vi "AlliGator Load FLIMbox Data v0.3.vi"(8 "Error In":errorcluster, 9 "Append":bool, 10 "FLIMbox Data in":T1 {"Base Frequency" min=-2147483648000000.0 max=2147483647000000.0}, 11 "File Path":path) -> (0 "Error Out":errorcluster, 2 "FLIMbox Data out":T1 {"Base Frequency" min=-2147483648000000.0 max=2147483647000000.0})   [LabVIEW 2021, in "AlliGator Files.lvlib"]
doc: "Loads FLIMBox dataset."
uses:
  AlliGator/AlliGator Files.lvlib
  FLIMbox Data.ctl
  FLIMbox Harmonic Data.ctl
  <vilib>/addons/h5labview2/base/lib_path.vi
  <vilib>/addons/h5labview2/base/H5Equery.vi
  <vilib>/addons/h5labview2/base/hid_t.ctl
  <vilib>/addons/h5labview2/dataset/H5Dread.llb/H5Dread.xnode
  <vilib>/addons/h5labview2/file/H5F.lvlib
  Time/Time.lvlib
  FLIMBox.lvlib
  <vilib>/addons/h5labview2/group/H5G.lvlib
panel:
  # "see the AlliGator License on the block diagram (Ctrl+E or Window:Show Block Diagram)"
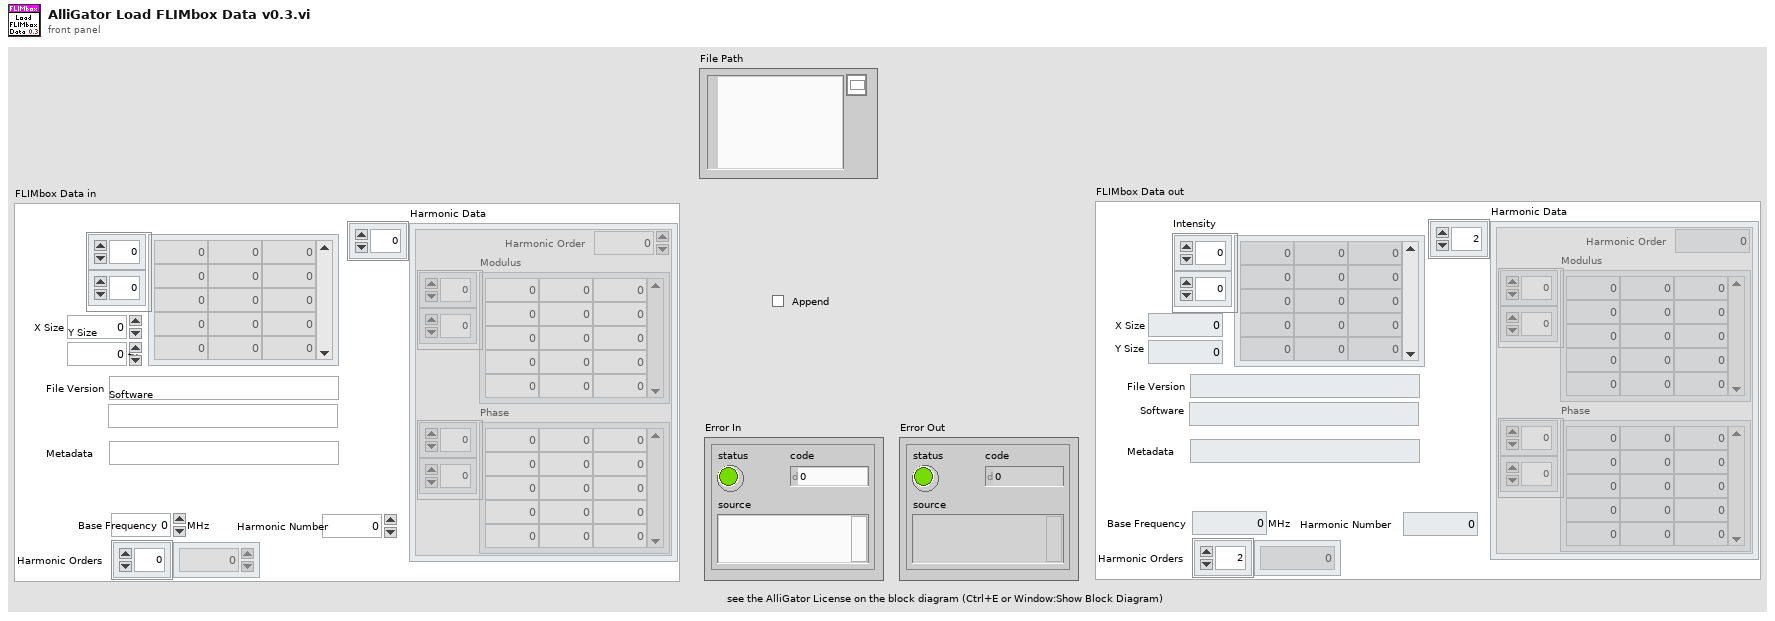
[diagram p1: front panel]
types:
  T1 = typedef "FLIMBox.lvlib/FLIMbox Data.ctl" = cluster{"Software":string, "Base Frequency":dbl[unit], "X Size":i32, "Y Size":i32, "Metadata":string, "Intensity":sgl[][], "Harmonic Number":u8, "Harmonic Orders":u8[], "Harmonic Data":T2[], "File Version":string}
  T2 = typedef "FLIMBox.lvlib/FLIMbox Harmonic Data.ctl" = cluster{"Modulus":sgl[][], "Phase":sgl[][], "Harmonic Order":u8}
  T3 = typedef "hid_t.ctl" = i64
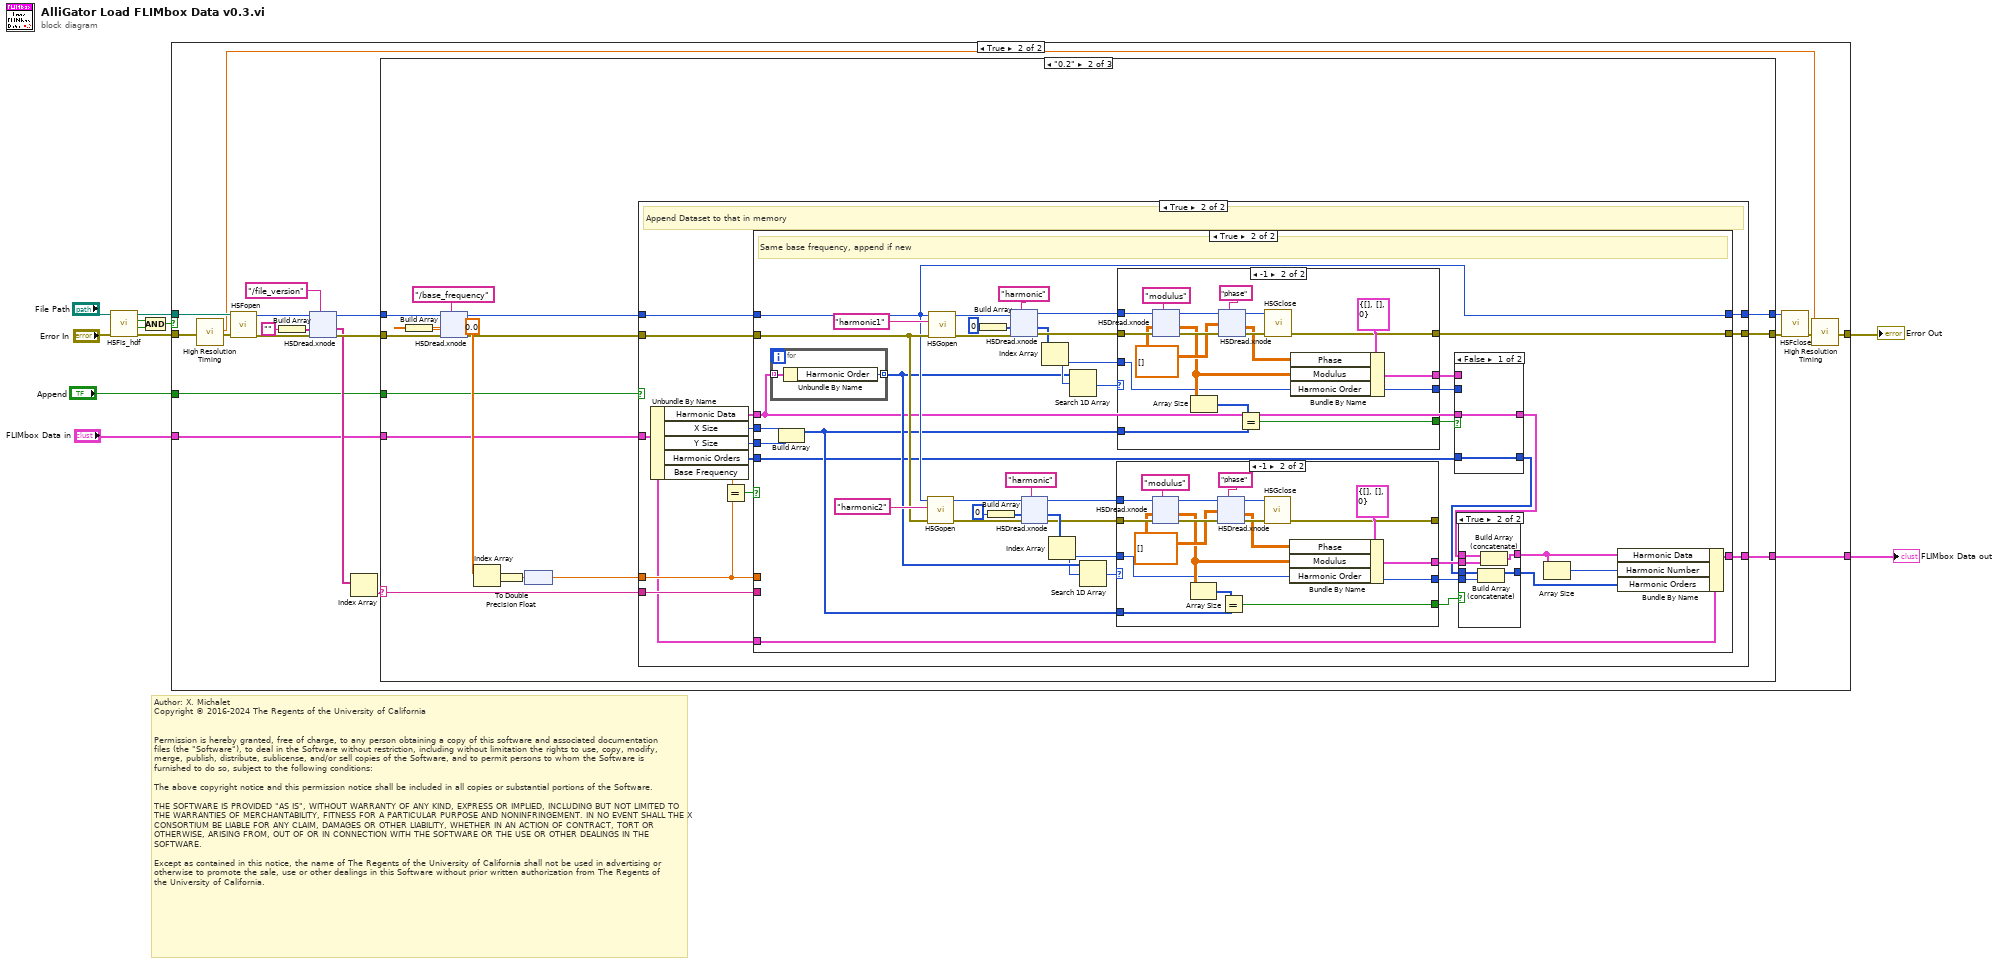
[diagram p0: block diagram]
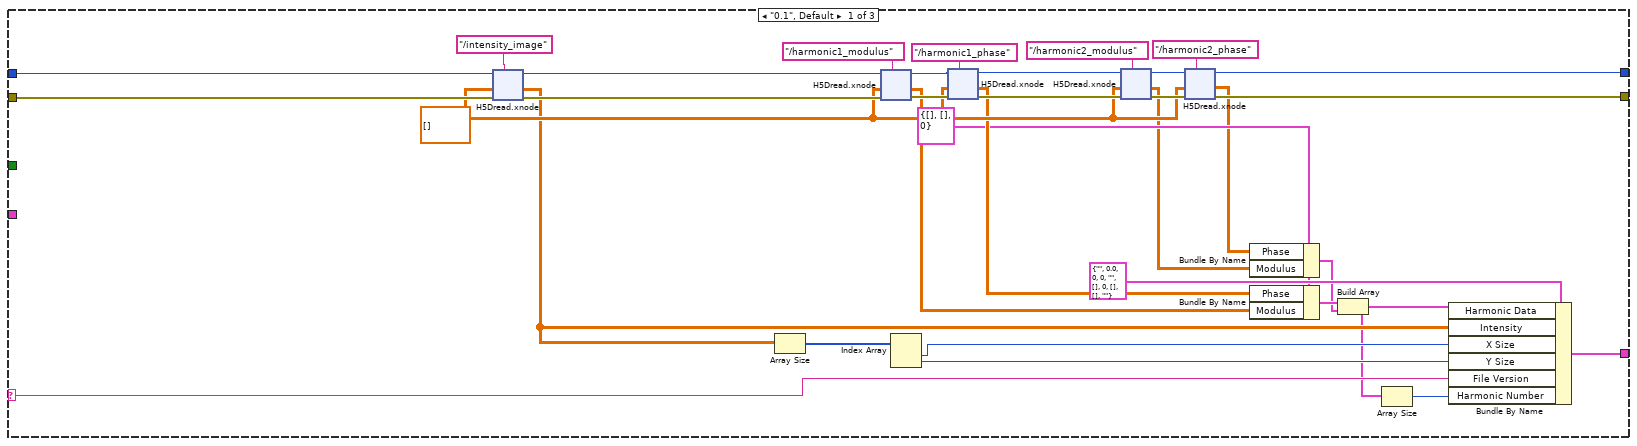
[diagram p3: hidden frame]
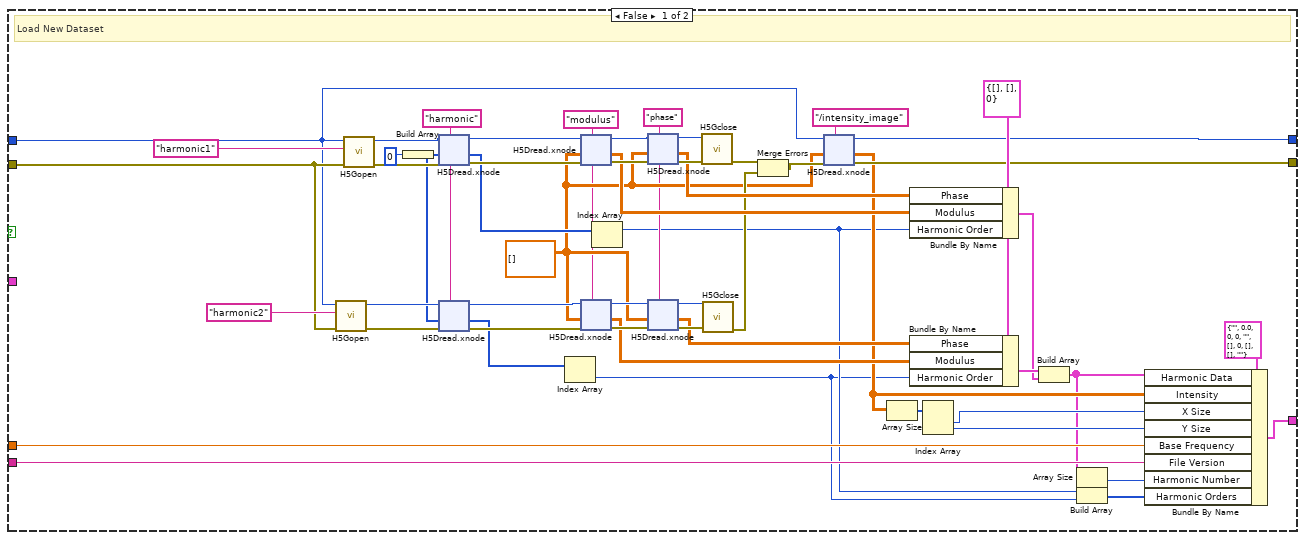
[diagram p4: hidden frame]
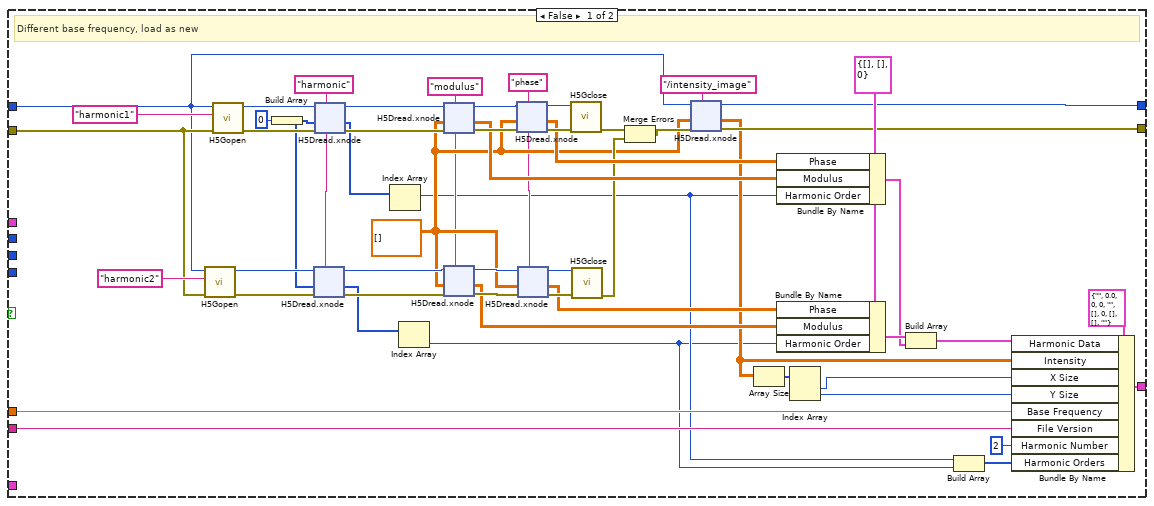
[diagram p5: hidden frame]
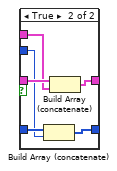
[diagram p7: hidden frame]
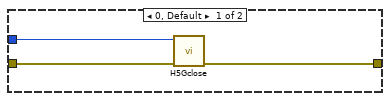
[diagram p8: hidden frame]
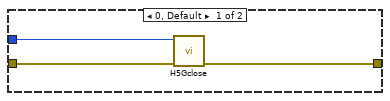
[diagram p9: hidden frame]
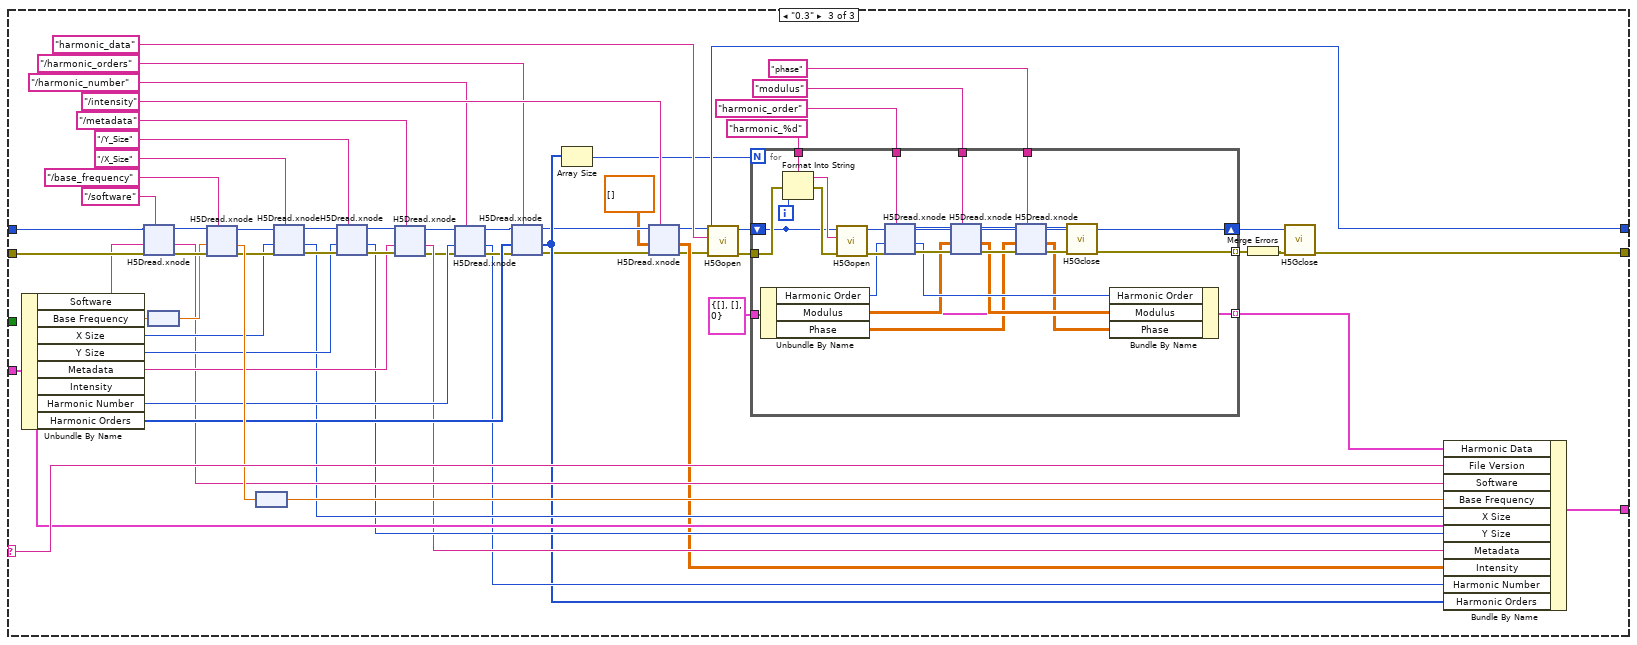
[diagram p10: hidden frame]
diagram:
  # "Author: X. Michalet\nCopyright © 2016-2024 The Regents of the University of California\n \n\nPermission is hereby granted, free of charge, to any person obtaining a copy of this software and associated documentation files (the \"Software\"), to deal in the Software without restriction, including without limitation the rights to use, copy, modify, merge, publish, distribute, sublicense, and/or sell copies of the Software, and to permit persons to whom the Software is furnished to do so, subject to the following conditions:\n\nThe above copyright notice and this permission notice shall be included in all copies or substantial portions of the Software.\n\nTHE SOFTWARE IS PROVIDED \"AS IS\", WITHOUT WARRANTY OF ANY KIND, EXPRESS OR IMPLIED, INCLUDING BUT NOT LIMITED TO THE WARRANTIES OF MERCHANTABILITY, FITNESS FOR A PARTICULAR PURPOSE AND NONINFRINGEMENT. IN NO EVENT SHALL THE X CONSORTIUM BE LIABLE FOR ANY CLAIM, DAMAGES OR OTHER LIABILITY, WHETHER IN AN ACTION OF CONTRACT, TORT OR OTHERWISE, ARISING FROM, OUT OF OR IN CONNECTION WITH THE SOFTWARE OR THE USE OR OTHER DEALINGS IN THE SOFTWARE.\n\nExcept as contained in this notice, the name of The Regents of the University of California shall not be used in advertising or otherwise to promote the sale, use or other dealings in this Software without prior written authorization from The Regents of the University of California."
  n1 = call <vilib>:"H5Fis_hdf.vi"("error in (no error)"="Error In", "path in"="File Path") -> ("error out"=w5:errorcluster, "valid?"=w10:bool, "exists?"=w11:bool, "path out"=w6:path)  [unwired: 6 in]
  n2 = And(x=w11, y=w10) -> (x .and. y?=w7:bool)
  n3 = case shown="True" w7 {
    tunnel: w6 -> [_ w31]
    tunnel: w5 -> [w12 w30]
    tunnel: [w12 w19] -> w4
    tunnel: [_ w20] -> w3
    tunnel: "FLIMbox Data in" -> [_ w14]
    tunnel: "Append" -> [_ w13]
    frame False {
    }
    frame True {
      n4 = call "High Resolution Timing.vi"("Error In"=w30) -> ("elapsed (relative) seconds"=w18:dbl, "Error Out"=w32:errorcluster)  [unwired: 16 in, 1 out]
      n5 = call <vilib>:"H5Fopen.vi"("error in (no error)"=w32, "path"=w31) -> ("error out"=w24:errorcluster, "ref out"=w29:T3)  [unwired: 8 in]
      n6 = Build Array("") -> (w17:string[])
      n7 = xnode "H5Dread.xnode"("dataset name (this)"="/file_version", "error in (no error)"=w24, "default"=w17, "ref in"=w29) -> ("error out"=w25:errorcluster, "data"=w15:string[], "ref out"=w26:T3)  [unwired: 2 in, 1 out]
      n8 = Index Array(array=w15) -> (element=w16:string)  [unwired: 1 in]
      n9 = case shown="\"0.2\"" w16 {
        selector: w16 -> [w57 w172 w773]
        tunnel: w26 -> [w81 w170 w769]
        tunnel: w25 -> [w79 w171 w768]
        tunnel: [w65 w162 w724] -> w23
        tunnel: [w64 w160 w717] -> w21
        tunnel: [w58 w173 w774] -> w20
        tunnel: w14 -> [_ w158 w741]
        tunnel: w13 -> [_ w159 _]
        frame "0.1", Default {
          w54 = T2 {"Modulus"=[], "Phase"=[], "Harmonic Order"=0} ("Harmonic Data")
          w66 = sgl[][] [] ("Data")
          n10 = xnode "H5Dread.xnode"("dataset name (this)"="/intensity_image", "error in (no error)"=w79, "default"=w66, "ref in"=w81) -> ("error out"=w78:errorcluster, "data"=w62:sgl[][], "ref out"=w77:T3)  [unwired: 2 in, 1 out]
          n11 = Array Size(array=w62) -> (size(s)=w61:i32[])
          n12 = xnode "H5Dread.xnode"("dataset name (this)"="/harmonic1_modulus", "error in (no error)"=w78, "default"=w66, "ref in"=w77) -> ("error out"=w74:errorcluster, "data"=w56:sgl[][], "ref out"=w75:T3)  [unwired: 2 in, 1 out]
          n13 = Index Array(array=w61) -> (element #1=w60:i32, element #2=w59:i32)  [unwired: 2 in]
          n14 = xnode "H5Dread.xnode"("dataset name (this)"="/harmonic1_phase", "error in (no error)"=w74, "default"=w66, "ref in"=w75) -> ("error out"=w68:errorcluster, "data"=w55:sgl[][], "ref out"=w67:T3)  [unwired: 2 in, 1 out]
          n15 = xnode "H5Dread.xnode"("dataset name (this)"="/harmonic2_modulus", "error in (no error)"=w68, "default"=w66, "ref in"=w67) -> ("error out"=w71:errorcluster, "data"=w52:sgl[][], "ref out"=w70:T3)  [unwired: 2 in, 1 out]
          n16 = xnode "H5Dread.xnode"("dataset name (this)"="/harmonic2_phase", "error in (no error)"=w71, "default"=w66, "ref in"=w70) -> ("error out"=w65:errorcluster, "data"=w53:sgl[][], "ref out"=w64:T3)  [unwired: 2 in, 1 out]
          n17 = Bundle By Name(cluster=w54, "Phase"=w53, "Modulus"=w52) -> (w50:T2)
          n18 = Bundle By Name(cluster=w54, "Phase"=w55, "Modulus"=w56) -> (w51:T2)
          n19 = Build Array(w51, w50) -> (w49:T2[])
          n20 = Array Size(array=w49) -> (size(s)=w48:i32)
          n21 = Bundle By Name(cluster=T1 {"Software"="", "Base Frequency"=0.0, "X Size"=0, "Y Size"=0, "Metadata"="", "Intensity"=[], "Harmonic Number"=0, "Harmonic Orders"=[], "Harmonic Data"=[], "File Version"=""} ("Data"), "Harmonic Data"=w49, "Intensity"=w62, "X Size"=w60, "Y Size"=w59, "File Version"=w57, "Harmonic Number"=w48) -> (w58:T1)
        }
        frame "0.2" {
          n22 = Build Array(sgl 0.0 ("U32")) -> (w165:sgl[])
          n23 = xnode "H5Dread.xnode"("dataset name (this)"="/base_frequency", "error in (no error)"=w171, "default"=w165, "ref in"=w170) -> ("error out"=w163:errorcluster, "data"=w167:sgl[], "ref out"=w161:T3)  [unwired: 2 in, 1 out]
          n24 = Index Array(array=w167) -> (element=w164:sgl)  [unwired: 1 in]
          n25 = To Double Precision Float(number=w164) -> (double precision float=w157:dbl)
          n26 = node(w157) -> (w166:dbl[unit])
          n27 = case shown="True" w159 {
            tunnel: [w234 w361] -> w173
            tunnel: w172 -> [w233 w360]
            tunnel: w166 -> [w229 w354]
            tunnel: w163 -> [w205 w359]
            tunnel: [w203 w358] -> w162
            tunnel: w161 -> [w201 w357]
            tunnel: [w200 w356] -> w160
            tunnel: w158 -> [_ w349]
            frame False {
              w194 = "harmonic" ("dataset name (this)")
              w232 = T2 {"Modulus"=[], "Phase"=[], "Harmonic Order"=0} ("Harmonic Data")
              w196 = "phase" ("dataset name (this)")
              w195 = "modulus" ("dataset name (this)")
              w199 = sgl[][] [] ("Data")
              # "Load New Dataset"
              n28 = call <vilib>:"H5Gopen.vi"("error in (no error)"=w205, "name"="harmonic2" ("dataset name (this)"), "ref in"=w201) -> ("error out"=w213:errorcluster, "group out"=w212:T3)  [unwired: 7 in]
              n29 = call <vilib>:"H5Gopen.vi"("error in (no error)"=w205, "name"="harmonic1" ("dataset name (this)"), "ref in"=w201) -> ("error out"=w220:errorcluster, "group out"=w219:T3)  [unwired: 7 in]
              n30 = Build Array(u8 0 ("Harmonic Order")) -> (w197:u8[])
              n31 = xnode "H5Dread.xnode"("dataset name (this)"=w194, "error in (no error)"=w220, "default"=w197, "ref in"=w219) -> ("error out"=w228:errorcluster, "data"=w225:u8[], "ref out"=w227:T3)  [unwired: 2 in, 1 out]
              n32 = xnode "H5Dread.xnode"("dataset name (this)"=w194, "error in (no error)"=w213, "default"=w197, "ref in"=w212) -> ("error out"=w224:errorcluster, "data"=w222:u8[], "ref out"=w223:T3)  [unwired: 2 in, 1 out]
              n33 = Index Array(array=w222) -> (element=w190:u8)  [unwired: 1 in]
              n34 = xnode "H5Dread.xnode"("dataset name (this)"=w195, "error in (no error)"=w228, "default"=w199, "ref in"=w227) -> ("error out"=w241:errorcluster, "data"=w215:sgl[][], "ref out"=w242:T3)  [unwired: 2 in, 1 out]
              n35 = xnode "H5Dread.xnode"("dataset name (this)"=w195, "error in (no error)"=w224, "default"=w199, "ref in"=w223) -> ("error out"=w240:errorcluster, "data"=w206:sgl[][], "ref out"=w239:T3)  [unwired: 2 in, 1 out]
              n36 = Index Array(array=w225) -> (element=w191:u8)  [unwired: 1 in]
              n37 = xnode "H5Dread.xnode"("dataset name (this)"=w196, "error in (no error)"=w241, "default"=w199, "ref in"=w242) -> ("error out"=w218:errorcluster, "data"=w216:sgl[][], "ref out"=w217:T3)  [unwired: 2 in, 1 out]
              n38 = xnode "H5Dread.xnode"("dataset name (this)"=w196, "error in (no error)"=w240, "default"=w199, "ref in"=w239) -> ("error out"=w210:errorcluster, "data"=w207:sgl[][], "ref out"=w211:T3)  [unwired: 2 in, 1 out]
              n39 = call <vilib>:"H5Gclose.vi"("error in (no error)"=w218, "group in"=w217) -> ("error out"=w209:errorcluster)  [unwired: 9 in]
              n40 = call <vilib>:"H5Gclose.vi"("error in (no error)"=w210, "group in"=w211) -> ("error out"=w208:errorcluster)  [unwired: 9 in]
              n41 = Merge Errors(w209, w208) -> (w204:errorcluster)
              n42 = xnode "H5Dread.xnode"("dataset name (this)"="/intensity_image", "error in (no error)"=w204, "default"=w199, "ref in"=w201) -> ("error out"=w203:errorcluster, "data"=w198:sgl[][], "ref out"=w200:T3)  [unwired: 2 in, 1 out]
              n43 = Array Size(array=w198) -> (size(s)=w237:i32[])
              n44 = Bundle By Name(cluster=w232, "Phase"=w216, "Modulus"=w215, "Harmonic Order"=w191) -> (w230:T2)
              n45 = Bundle By Name(cluster=w232, "Phase"=w207, "Modulus"=w206, "Harmonic Order"=w190) -> (w231:T2)
              n46 = Index Array(array=w237) -> (element #1=w236:i32, element #2=w235:i32)  [unwired: 2 in]
              n47 = Build Array(w231, w230) -> (w193:T2[])
              n48 = Array Size(array=w193) -> (size(s)=w192:i32)
              n49 = Build Array(w191, w190) -> (w189:u8[])
              n50 = Bundle By Name(cluster=T1 {"Software"="", "Base Frequency"=0.0, "X Size"=0, "Y Size"=0, "Metadata"="", "Intensity"=[], "Harmonic Number"=0, "Harmonic Orders"=[], "Harmonic Data"=[], "File Version"=""} ("Data"), "Harmonic Data"=w193, "Intensity"=w198, "X Size"=w236, "Y Size"=w235, "Base Frequency"=w229, "File Version"=w233, "Harmonic Number"=w192, "Harmonic Orders"=w189) -> (w234:T1)
            }
            frame True {
              # "Append Dataset to that in memory"
              n51 = Unbundle By Name(w349) -> ("Harmonic Data"=w352:T2[], "X Size"=w351:i32, "Y Size"=w350:i32, "Harmonic Orders"=w348:u8[], "Base Frequency"=w355:dbl[unit])
              n52 = Equal?(x=w355, y=w354) -> (x = y?=w353:bool)
              n53 = case shown="True" w353 {
                tunnel: [w407 w564] -> w361
                tunnel: w360 -> [w406 _]
                tunnel: w359 -> [w378 w547]
                tunnel: [w376 w545] -> w358
                tunnel: w357 -> [w374 w546]
                tunnel: [w373 w546] -> w356
                tunnel: w354 -> [w370 _]
                tunnel: w352 -> [_ w533]
                tunnel: w351 -> [_ w541]
                tunnel: w350 -> [_ w542]
                tunnel: w349 -> [_ w528]
                tunnel: w348 -> [_ w525]
                frame False {
                  w367 = "harmonic" ("dataset name (this)")
                  w405 = T2 {"Modulus"=[], "Phase"=[], "Harmonic Order"=0} ("Harmonic Data")
                  w369 = "phase" ("dataset name (this)")
                  w368 = "modulus" ("dataset name (this)")
                  w372 = sgl[][] [] ("Data")
                  # "Different base frequency, load as new"
                  n54 = call <vilib>:"H5Gopen.vi"("error in (no error)"=w378, "name"="harmonic2" ("dataset name (this)"), "ref in"=w374) -> ("error out"=w386:errorcluster, "group out"=w385:T3)  [unwired: 7 in]
                  n55 = call <vilib>:"H5Gopen.vi"("error in (no error)"=w378, "name"="harmonic1" ("dataset name (this)"), "ref in"=w374) -> ("error out"=w393:errorcluster, "group out"=w392:T3)  [unwired: 7 in]
                  n56 = Build Array(u8 0 ("Harmonic Order")) -> (w366:u8[])
                  n57 = xnode "H5Dread.xnode"("dataset name (this)"=w367, "error in (no error)"=w386, "default"=w366, "ref in"=w385) -> ("error out"=w397:errorcluster, "data"=w395:u8[], "ref out"=w396:T3)  [unwired: 2 in, 1 out]
                  n58 = xnode "H5Dread.xnode"("dataset name (this)"=w367, "error in (no error)"=w393, "default"=w366, "ref in"=w392) -> ("error out"=w401:errorcluster, "data"=w398:u8[], "ref out"=w400:T3)  [unwired: 2 in, 1 out]
                  n59 = Index Array(array=w398) -> (element=w364:u8)  [unwired: 1 in]
                  n60 = Index Array(array=w395) -> (element=w363:u8)  [unwired: 1 in]
                  n61 = xnode "H5Dread.xnode"("dataset name (this)"=w368, "error in (no error)"=w401, "default"=w372, "ref in"=w400) -> ("error out"=w414:errorcluster, "data"=w388:sgl[][], "ref out"=w415:T3)  [unwired: 2 in, 1 out]
                  n62 = xnode "H5Dread.xnode"("dataset name (this)"=w368, "error in (no error)"=w397, "default"=w372, "ref in"=w396) -> ("error out"=w413:errorcluster, "data"=w379:sgl[][], "ref out"=w412:T3)  [unwired: 2 in, 1 out]
                  n63 = xnode "H5Dread.xnode"("dataset name (this)"=w369, "error in (no error)"=w414, "default"=w372, "ref in"=w415) -> ("error out"=w391:errorcluster, "data"=w389:sgl[][], "ref out"=w390:T3)  [unwired: 2 in, 1 out]
                  n64 = xnode "H5Dread.xnode"("dataset name (this)"=w369, "error in (no error)"=w413, "default"=w372, "ref in"=w412) -> ("error out"=w383:errorcluster, "data"=w380:sgl[][], "ref out"=w384:T3)  [unwired: 2 in, 1 out]
                  n65 = call <vilib>:"H5Gclose.vi"("error in (no error)"=w391, "group in"=w390) -> ("error out"=w382:errorcluster)  [unwired: 9 in]
                  n66 = call <vilib>:"H5Gclose.vi"("error in (no error)"=w383, "group in"=w384) -> ("error out"=w381:errorcluster)  [unwired: 9 in]
                  n67 = Merge Errors(w382, w381) -> (w377:errorcluster)
                  n68 = xnode "H5Dread.xnode"("dataset name (this)"="/intensity_image", "error in (no error)"=w377, "default"=w372, "ref in"=w374) -> ("error out"=w376:errorcluster, "data"=w371:sgl[][], "ref out"=w373:T3)  [unwired: 2 in, 1 out]
                  n69 = Array Size(array=w371) -> (size(s)=w410:i32[])
                  n70 = Bundle By Name(cluster=w405, "Phase"=w389, "Modulus"=w388, "Harmonic Order"=w364) -> (w403:T2)
                  n71 = Bundle By Name(cluster=w405, "Phase"=w380, "Modulus"=w379, "Harmonic Order"=w363) -> (w404:T2)
                  n72 = Index Array(array=w410) -> (element #1=w409:i32, element #2=w408:i32)  [unwired: 2 in]
                  n73 = Build Array(w404, w403) -> (w402:T2[])
                  n74 = Build Array(w364, w363) -> (w362:u8[])
                  n75 = Bundle By Name(cluster=T1 {"Software"="", "Base Frequency"=0.0, "X Size"=0, "Y Size"=0, "Metadata"="", "Intensity"=[], "Harmonic Number"=0, "Harmonic Orders"=[], "Harmonic Data"=[], "File Version"=""} ("Data"), "Harmonic Data"=w402, "Intensity"=w371, "X Size"=w409, "Y Size"=w408, "Base Frequency"=w370, "File Version"=w406, "Harmonic Number"=u8 2, "Harmonic Orders"=w362) -> (w407:T1)
                }
                frame True {
                  # "Same base frequency, append if new"
                  n76 = for {
                    tunnel: w533 -> [w714] mode=indexing
                    tunnel: [w713] -> w538 mode=indexing
                    n77 = Unbundle By Name(w714) -> ("Harmonic Order"=w713:u8)
                  }
                  n78 = Build Array(w541, w542) -> (w536:i32[])
                  n79 = call <vilib>:"H5Gopen.vi"("error in (no error)"=w547, "name"="harmonic2" ("dataset name (this)"), "ref in"=w546) -> ("error out"=w549:errorcluster, "group out"=w548:T3)  [unwired: 7 in]
                  n80 = call <vilib>:"H5Gopen.vi"("error in (no error)"=w547, "name"="harmonic1" ("dataset name (this)"), "ref in"=w546) -> ("error out"=w552:errorcluster, "group out"=w551:T3)  [unwired: 7 in]
                  n81 = Build Array(u8 0 ("Harmonic Order")) -> (w556:u8[])
                  n82 = Build Array(u8 0 ("Harmonic Order")) -> (w555:u8[])
                  n83 = xnode "H5Dread.xnode"("dataset name (this)"="harmonic", "error in (no error)"=w552, "default"=w556, "ref in"=w551) -> ("error out"=w563:errorcluster, "data"=w560:u8[], "ref out"=w562:T3)  [unwired: 2 in, 1 out]
                  n84 = xnode "H5Dread.xnode"("dataset name (this)"="harmonic", "error in (no error)"=w549, "default"=w555, "ref in"=w548) -> ("error out"=w540:errorcluster, "data"=w557:u8[], "ref out"=w539:T3)  [unwired: 2 in, 1 out]
                  n85 = Index Array(array=w560) -> (element=w543:u8)  [unwired: 1 in]
                  n86 = Index Array(array=w557) -> (element=w535:u8)  [unwired: 1 in]
                  n87 = Search 1D Array(1D array=w538, element=w543) -> (index of element=w544:i32)  [unwired: 1 in]
                  n88 = Search 1D Array(1D array=w538, element=w535) -> (index of element=w537:i32)  [unwired: 1 in]
                  n89 = case shown="-1" w537 {
                    tunnel: [_ w626] -> w529
                    tunnel: w540 -> [w613 w625]
                    tunnel: w539 -> [w612 w624]
                    tunnel: [w611 w619] -> _
                    tunnel: w536 -> [_ w616]
                    tunnel: [_ w615] -> w531
                    tunnel: w535 -> [_ w614]
                    tunnel: [_ w614] -> w522
                    frame 0, Default {
                      n90 = call <vilib>:"H5Gclose.vi"("error in (no error)"=w613, "group in"=w612) -> ("error out"=w611:errorcluster)  [unwired: 9 in]
                    }
                    frame -1 {
                      w620 = sgl[][] [] ("Data")
                      n91 = xnode "H5Dread.xnode"("dataset name (this)"="modulus", "error in (no error)"=w625, "default"=w620, "ref in"=w624) -> ("error out"=w629:errorcluster, "data"=w618:sgl[][], "ref out"=w630:T3)  [unwired: 2 in, 1 out]
                      n92 = Array Size(array=w618) -> (size(s)=w617:i32[])
                      n93 = xnode "H5Dread.xnode"("dataset name (this)"="phase", "error in (no error)"=w629, "default"=w620, "ref in"=w630) -> ("error out"=w623:errorcluster, "data"=w621:sgl[][], "ref out"=w622:T3)  [unwired: 2 in, 1 out]
                      n94 = Equal?(x=w617, y=w616) -> (x = y?=w615:bool)
                      n95 = call <vilib>:"H5Gclose.vi"("error in (no error)"=w623, "group in"=w622) -> ("error out"=w619:errorcluster)  [unwired: 9 in]
                      n96 = Bundle By Name(cluster=T2 {"Modulus"=[], "Phase"=[], "Harmonic Order"=0} ("Harmonic Data"), "Phase"=w621, "Modulus"=w618, "Harmonic Order"=w614) -> (w626:T2)
                    }
                  }
                  n97 = case shown="-1" w544 {
                    tunnel: [_ w677] -> w532
                    tunnel: w563 -> [w664 w676]
                    tunnel: w562 -> [w663 w675]
                    tunnel: [w662 w670] -> w545
                    tunnel: w543 -> [_ w665]
                    tunnel: w536 -> [_ w667]
                    tunnel: [_ w666] -> w534
                    tunnel: [_ w665] -> w524
                    frame 0, Default {
                      n98 = call <vilib>:"H5Gclose.vi"("error in (no error)"=w664, "group in"=w663) -> ("error out"=w662:errorcluster)  [unwired: 9 in]
                    }
                    frame -1 {
                      w671 = sgl[][] [] ("Data")
                      n99 = xnode "H5Dread.xnode"("dataset name (this)"="modulus", "error in (no error)"=w676, "default"=w671, "ref in"=w675) -> ("error out"=w680:errorcluster, "data"=w669:sgl[][], "ref out"=w681:T3)  [unwired: 2 in, 1 out]
                      n100 = Array Size(array=w669) -> (size(s)=w668:i32[])
                      n101 = xnode "H5Dread.xnode"("dataset name (this)"="phase", "error in (no error)"=w680, "default"=w671, "ref in"=w681) -> ("error out"=w674:errorcluster, "data"=w672:sgl[][], "ref out"=w673:T3)  [unwired: 2 in, 1 out]
                      n102 = Equal?(x=w668, y=w667) -> (x = y?=w666:bool)
                      n103 = call <vilib>:"H5Gclose.vi"("error in (no error)"=w674, "group in"=w673) -> ("error out"=w670:errorcluster)  [unwired: 9 in]
                      n104 = Bundle By Name(cluster=T2 {"Modulus"=[], "Phase"=[], "Harmonic Order"=0} ("Harmonic Data"), "Phase"=w672, "Modulus"=w669, "Harmonic Order"=w665) -> (w677:T2)
                    }
                  }
                  n105 = case shown="False" w534 {
                    tunnel: w533 -> [w604 w610]
                    tunnel: w532 -> [_ w609]
                    tunnel: [w604 w608] -> w530
                    tunnel: w525 -> [w603 w607]
                    tunnel: w524 -> [_ w606]
                    tunnel: [w603 w605] -> w523
                    frame False {
                    }
                    frame True {
                      n106 = Build Array (concatenate)(w607, w606) -> (w605:u8[])
                      n107 = Build Array (concatenate)(w610, w609) -> (w608:T2[])
                    }
                  }
                  n108 = case shown="True" w531 {
                    tunnel: w530 -> [w596 w602]
                    tunnel: w529 -> [_ w601]
                    tunnel: [w596 w600] -> w527
                    tunnel: w523 -> [w595 w599]
                    tunnel: w522 -> [_ w598]
                    tunnel: [w595 w597] -> w521
                    frame False {
                    }
                    frame True {
                      n109 = Build Array (concatenate)(w599, w598) -> (w597:u8[])
                      n110 = Build Array (concatenate)(w602, w601) -> (w600:T2[])
                    }
                  }
                  n111 = Array Size(array=w527) -> (size(s)=w526:i32)
                  n112 = Bundle By Name(cluster=w528, "Harmonic Data"=w527, "Harmonic Number"=w526, "Harmonic Orders"=w521) -> (w564:T1)
                }
              }
            }
          }
        }
        frame "0.3" {
          n113 = Unbundle By Name(w741) -> ("Software"=w764:string, "Base Frequency"=w763:dbl[unit], "X Size"=w760:i32, "Y Size"=w757:i32, "Metadata"=w753:string, "Harmonic Number"=w750:u8, "Harmonic Orders"=w749:u8[])  [unwired: 1 out]
          n114 = xnode "H5Dread.xnode"("dataset name (this)"="/software", "error in (no error)"=w768, "default"=w764, "ref in"=w769) -> ("data"=w740:string, "ref out"=w766:T3)  [unwired: 2 in, 2 out]
          n115 = node(w763) -> (w762:dbl)
          n116 = xnode "H5Dread.xnode"("dataset name (this)"="/base_frequency", "error in (no error)"=w768, "default"=w762, "ref in"=w766) -> ("error out"=w761:errorcluster, "data"=w770:dbl, "ref out"=w746:T3)  [unwired: 2 in, 1 out]
          n117 = node(w770) -> (w739:dbl[unit])
          n118 = xnode "H5Dread.xnode"("dataset name (this)"="/X_Size", "error in (no error)"=w761, "default"=w760, "ref in"=w746) -> ("error out"=w758:errorcluster, "data"=w738:i32, "ref out"=w745:T3)  [unwired: 2 in, 1 out]
          n119 = xnode "H5Dread.xnode"("dataset name (this)"="/Y_Size", "error in (no error)"=w758, "default"=w757, "ref in"=w745) -> ("error out"=w755:errorcluster, "data"=w737:i32, "ref out"=w744:T3)  [unwired: 2 in, 1 out]
          n120 = xnode "H5Dread.xnode"("dataset name (this)"="/metadata", "error in (no error)"=w755, "default"=w753, "ref in"=w744) -> ("error out"=w721:errorcluster, "data"=w736:string, "ref out"=w722:T3)  [unwired: 2 in, 1 out]
          n121 = xnode "H5Dread.xnode"("dataset name (this)"="/harmonic_number", "error in (no error)"=w721, "default"=w750, "ref in"=w722) -> ("error out"=w748:errorcluster, "data"=w734:u8, "ref out"=w743:T3)  [unwired: 2 in, 1 out]
          n122 = xnode "H5Dread.xnode"("dataset name (this)"="/harmonic_orders", "error in (no error)"=w748, "default"=w749, "ref in"=w743) -> ("error out"=w720:errorcluster, "data"=w733:u8[], "ref out"=w718:T3)  [unwired: 2 in, 1 out]
          n123 = Array Size(array=w733) -> (size(s)=w715:i32)
          n124 = xnode "H5Dread.xnode"("dataset name (this)"="/intensity", "error in (no error)"=w720, "default"=sgl[][] [] ("Intensity"), "ref in"=w718) -> ("error out"=w719:errorcluster, "data"=w735:sgl[][], "ref out"=w717:T3)  [unwired: 2 in, 1 out]
          n125 = call <vilib>:"H5Gopen.vi"("error in (no error)"=w719, "name"="harmonic_data" ("dataset name (this)"), "ref in"=w717) -> ("error out"=w772:errorcluster, "group out"=w771:T3)  [unwired: 7 in]
          n126 = for {
            N: w715 -> [_]
            tunnel: w772 -> [w910]
            shift-right: [w895] -> w725
            shift-left: w771 -> [w895]
            tunnel: "harmonic_%d" ("dataset name (this)") -> [w913]
            tunnel: "harmonic_order" ("dataset name (this)") -> [w907]
            tunnel: T2 {"Modulus"=[], "Phase"=[], "Harmonic Order"=0} ("Harmonic Data") -> [w901]
            tunnel: "modulus" ("dataset name (this)") -> [w903]
            tunnel: "phase" ("dataset name (this)") -> [w899]
            tunnel: [w897] -> w723 mode=indexing
            tunnel: [w896] -> w727 mode=indexing
            i -> [w914]
            n127 = Unbundle By Name(w901) -> ("Harmonic Order"=w906:u8, "Modulus"=w904:sgl[][], "Phase"=w900:sgl[][])
            n128 = Format Into String(format string=w913, error in=w910, w914) -> (resulting string=w912:string, error out=w911:errorcluster)  [unwired: 1 in]
            n129 = call <vilib>:"H5Gopen.vi"("error in (no error)"=w911, "name"=w912, "ref in"=w895) -> ("error out"=w909:errorcluster, "group out"=w908:T3)  [unwired: 7 in]
            n130 = xnode "H5Dread.xnode"("dataset name (this)"=w907, "error in (no error)"=w909, "default"=w906, "ref in"=w908) -> ("error out"=w918:errorcluster, "data"=w905:u8, "ref out"=w917:T3)  [unwired: 2 in, 1 out]
            n131 = xnode "H5Dread.xnode"("dataset name (this)"=w903, "error in (no error)"=w918, "default"=w904, "ref in"=w917) -> ("error out"=w919:errorcluster, "data"=w902:sgl[][], "ref out"=w920:T3)  [unwired: 2 in, 1 out]
            n132 = xnode "H5Dread.xnode"("dataset name (this)"=w899, "error in (no error)"=w919, "default"=w900, "ref in"=w920) -> ("error out"=w916:errorcluster, "data"=w898:sgl[][], "ref out"=w915:T3)  [unwired: 2 in, 1 out]
            n133 = call <vilib>:"H5Gclose.vi"("error in (no error)"=w916, "group in"=w915) -> ("error out"=w896:errorcluster)  [unwired: 9 in]
            n134 = Bundle By Name(cluster=w901, "Harmonic Order"=w905, "Modulus"=w902, "Phase"=w898) -> (w897:T2)
          }
          n135 = Merge Errors(w727) -> (w726:errorcluster)
          n136 = call <vilib>:"H5Gclose.vi"("error in (no error)"=w726, "group in"=w725) -> ("error out"=w724:errorcluster)  [unwired: 9 in]
          n137 = Bundle By Name(cluster=w741, "Harmonic Data"=w723, "File Version"=w773, "Software"=w740, "Base Frequency"=w739, "X Size"=w738, "Y Size"=w737, "Metadata"=w736, "Intensity"=w735, "Harmonic Number"=w734, "Harmonic Orders"=w733) -> (w774:T1)
        }
      }
      n138 = call <vilib>:"H5Fclose.vi"("error in (no error)"=w23, "ref"=w21) -> ("error out"=w22:errorcluster)  [unwired: 9 in]
      n139 = call "High Resolution Timing.vi"("relative seconds (NaN)"=w18, "Error In"=w22) -> ("Error Out"=w19:errorcluster)  [unwired: 15 in, 2 out]
    }
  }
  "Error Out" <- w4
  "FLIMbox Data out" <- w3
